vi "Replace Children.vi"(8 "error in (no error)":errorcluster, 10 "New Children":refnum<class "Data Item.lvclass">[](array[class]), 11 "Attribute in":refnum<class "Attribute.lvclass">) -> (0 "error out":errorcluster, 3 "Attribute out":refnum<class "Attribute.lvclass">)   [LabVIEW 2018, in "VILab.lvlib" / "Attribute.lvclass"]
uses:
  Attribute.lvclass
  Data Item.lvclass
  Attribute.lvclass/Attribute.ctl
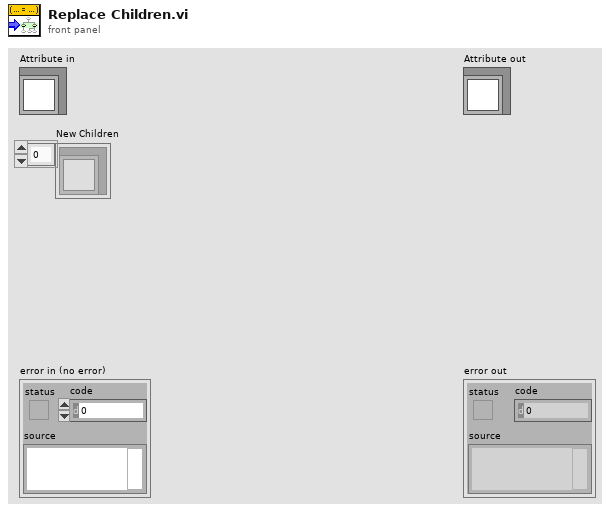
[diagram p1: front panel]
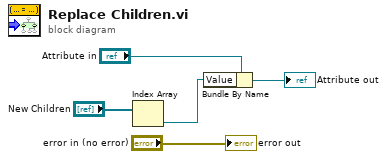
[diagram p0: block diagram]
diagram:
  n1 = Index Array(array="New Children") -> (element=w3:refnum<class "Data Item.lvclass">)  [unwired: 1 in]
  n2 = Bundle By Name(cluster="Attribute in", "Value"=w3) -> (→"Attribute out":refnum<class "Attribute.lvclass">)
  "error out" <- "error in (no error)"
